vi "comparison.vi"() -> ()   [LabVIEW 2019]
panel:
  out "In Range?":bool
  out "coerced(x)":dbl
  in  "x_input":dbl
  out "min(x,y)":i32
  out "max(x,y)":i32
  out "s? t:f":dbl
  in  "select":bool
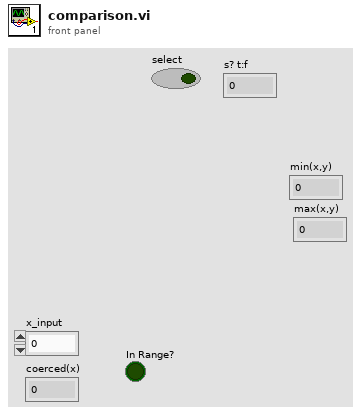
[diagram p1: front panel]
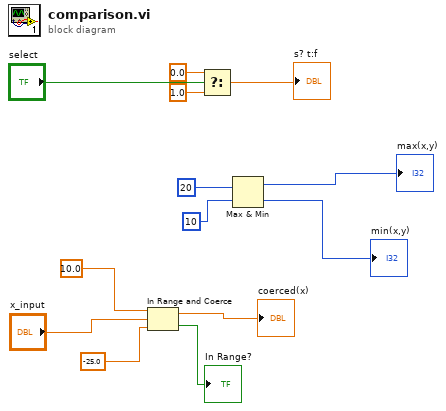
[diagram p0: block diagram]
diagram:
  n1 = In Range and Coerce(upper limit=10.0, x="x_input", lower limit=-25.0) -> (coerced(x)=→"coerced(x)":dbl, In Range?=→"In Range?":bool)
  n2 = Select(t=0.0, s="select", f=1.0) -> (s? t:f=→"s? t:f":dbl)
  n3 = Max & Min(x=20, y=10) -> (max(x,y)=→"max(x,y)":i32, min(x,y)=→"min(x,y)":i32)
